vi "ReadCapacity.vi"(11 "TypedCircularBuffer in":refnum<class "TypedCircularBuffer.lvclass">) -> (2 "capacity":u32, 3 "TypedCircularBuffer out":refnum<class "TypedCircularBuffer.lvclass">)   [LabVIEW 2024, in "TypedCircularBuffer.lvclass"]
uses:
  TypedCircularBuffer.lvclass
  TypedCircularBuffer.lvclass/TypedCircularBuffer.ctl
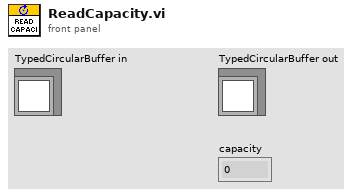
[diagram p1: front panel]
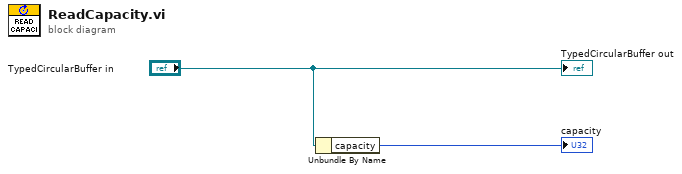
[diagram p0: block diagram]
diagram:
  n1 = Unbundle By Name("TypedCircularBuffer in") -> ("capacity"=→"capacity":u32)
  "TypedCircularBuffer out" <- "TypedCircularBuffer in"
